vi "ensterMF.vi"() -> ()   [LabVIEW 2019]
uses:
  <vilib>/Utility/error.llb/DialogType.ctl
  <vilib>/DAQmx/write.llb/DAQmx Write (Digital Bool 1Line 1Point).vi
  <vilib>/DAQmx/write.llb/DAQmx Write (Counter Frequency 1Chan 1Samp).vi
  <vilib>/DAQmx/miscellaneous.llb/DAQmx Fill In Error Info.vi
  <vilib>/DAQmx/create/channels.llb/DAQmx Create Channel (CO-Pulse Generation-Frequency).vi
  <vilib>/DAQmx/configure/timing.llb/DAQmx Timing (Implicit).vi
  <vilib>/addons/control/pid/pid.llb/PID (DBL).vi
  <vilib>/Utility/file.llb/Write Delimited Spreadsheet (string).vi
  <instrlib>/Agilent 34970/Agilent 34970.lvlib
  <resource>/objmgr/daqmx.rc
  <vilib>/addons/control/pid/NI_PID_pid.lvlib
  <instrlib>/Yokogawa WT200 Series/Yokogawa WT200 Series.lvlib
panel:
  in  "Tab Control":enum32{"Estufa", "Din", "ET_MF", "TPs", "T_Din"}(tab)
  in  "Ts":dbl=1.0
  out "Time":dbl=300.0 format="%<%H:%M:%S>t"
  in  "STOP":bool
  in  "Idenfier_Estufa":string="medsForno"
  in  "Estufa_ON":bool=TRUE
  in  "Frequency":dbl=1.0 format="%.6f"
  in  "PID gains":T1={"proportional gain (Kc)"=39.6, "integral time (Ti, min)"=14.617, "derivative time (Td, min)"=0.0} {"derivative time (Td, min)" format="%.3f"; "integral time (Ti, min)" format="%.3f"; "proportional gain (Kc)" format="%.6f"}
  out "Process variable and Setpoint":cluster{"initial PV":dbl, "SP:":dbl}(graph)
  out "MV":dbl(graph)
  in  "SP:":dbl(slide)=70.0 min=0.0 max=0.0 scale=25.0..70.0
  out "Temperature CH9 [degC]":dbl
  out "Temperature CH4 [degC]":dbl
  out "Iteration":i32
  out "Duty Cycle":sgl=0.1 min=0.1 max=99.9 format="%#_6f"
  out "PV":dbl
  in  "Tempo de integração (s)":u32=5 min=1 max=60 step=1
  out "Chart tensão numeric":cluster{"V(A)":dbl, "V(B)":dbl, "V(E)":dbl}(graph)={"V(A)"=0.0, "V(B)"=0.0, "V(E)"=228.25999450683594}
  out "Chart corrente numeric":cluster{"I(A)":dbl, "I(B)":dbl, "I(E)":dbl}(graph)={"I(A)"=0.0, "I(B)"=0.0, "I(E)"=0.14239999651908875}
  out "Chart potencia numeric":T2(graph)={"PC(A)"=0.0, "PC(B)"=7.200000254670158e-05, "PC(T)"=7.200000254670158e-05, "PL(A)"=0.0, "PL(B)"=0.0, "PL(T)"=0.0, "PC(E)"=1.0970638990402222, "PL(E)"=1.0099999904632568}
  in  "Realiza medição WT230":bool=TRUE
  in  "Medição contínua? WT230":bool=TRUE
  in  "Parâmetros serial":T3={"Serial VCC"="COM7", "timeout"=2, "baud rate"=600, "flow control"=0, "data bits"=8, "parity"=enum."None", "stop bits"=10, "termination char"=FALSE} {"stop bits" items=["1.0"=10, "1.5"=15, "2.0"=20]; "flow control" items=["None", "XON/XOFF", "RTS/CTS", "XON/XOFF & RTS/CTS", "DTR/DSR", "XON/XOFF & DTR/DSR"]}
  in  "Velocidade (RPM)":u16 min=1000 max=10000 step=100
  in  "Mensagem":T4(ring)=enum."Read power"
  in  "Limite de corrente":dbl=0.075 min=0.0 max=0.4 step=0.01 format="%.4f"
  in  "Limite de tensão":dbl=30.0 min=0.0 max=30.0 step=0.5 format="%.4f"
  in  "Seta carga":bool
  in  "Enviar velocidade":bool
  in  "Envia mensagem":bool
  in  "Parar motor":bool
  out "Tradução":string
  out "Resposta":string
  in  "Liga Fonte":bool
  out "watt num cluster":T5
  out "Corrente de saída":dbl format="%.4f"
  out "Tensão de saída":dbl format="%.4f"
  out "t":dbl
  out "PL(T)":dbl
  out "PC(T)":dbl
  out "PC(E)":dbl
  out "PL(E)":dbl
  in  "Identifier_Watt":string="medsWatt"
  in  "Idenfier_Freio":string="medsFreio"
  out "MV_I":dbl(graph)
  in  "PID gains MF":T1={"proportional gain (Kc)"=83.141, "integral time (Ti, min)"=1.0049, "derivative time (Td, min)"=0.0} {"derivative time (Td, min)" format="%.3f"; "integral time (Ti, min)" format="%.3f"; "proportional gain (Kc)" format="%.6f"}
  out "Grafico MF ENS":cluster{"initial PV":dbl, "SP:":dbl}(graph)
  out "MV_MF":sgl=0.1 min=0.1 max=99.9 format="%#_6f"
  out "PV_MF":dbl
  in  "Ts MF":dbl=1.0
  in  "Automatic":bool
  in  "SP_MF":dbl(slide)=69.0 caption="SP:" min=0.0 max=0.0 scale=25.0..70.0
  in  "Ident_EnsTerMF":string="medsETMF"
  in  "Tab Control 2":enum32{"1-7", "8-15"}(tab)
  out "G. TP 1":cluster{dbl, "index":i32}(graph)
  out "TP 1":dbl
  out "TP 2":dbl
  out "G. TP 2":cluster{dbl, "index":i32}(graph)
  out "G. TP 3":cluster{dbl, "index":i32}(graph)
  out "TP 3":dbl
  out "G. TP 5":cluster{dbl, "index":i32}(graph)
  out "TP 5":dbl
  out "G. TP 6":cluster{dbl, "index":i32}(graph)
  out "TP 6":dbl
  out "G. TP 7":cluster{dbl, "index":i32}(graph)
  out "TP 7":dbl
  out "G. TP 8":cluster{dbl, "index":i32}(graph)
  out "TP 8":dbl
  out "G. TP 10":cluster{dbl, "index":i32}(graph)
  out "TP 10":dbl
  out "G. TP 11":cluster{dbl, "index":i32}(graph)
  out "TP 11":dbl
  out "G. TP 12":cluster{dbl, "index":i32}(graph)
  out "TP 12":dbl
  out "G. TP 13":cluster{dbl, "index":i32}(graph)
  out "TP 13":dbl
  out "G. TP 15":cluster{dbl, "index":i32}(graph)
  out "TP 15":dbl
  in  "Idenfier_Ens. Term.":string="medsETMA"
  out "Chart Temperatura":cluster{dbl, dbl, dbl, dbl, dbl, dbl}(graph)={21.505, 22.941, 24.092, 23.94, 23.972, 20.648}
  out "temperature num cluster":T6
  # "Controle de Temperatura da Estufa"
  # "Geral"
  # "Respostas do Sistema em Malha Fechada"
  # "Controles"
  # "Medidas"
  # "Freio"
  # "Wattímetro WT230 Yokogawa"
  # "Controles:"
  # "Controles"
  # "Medidas"
  # "Respostas temporais"
  # "Medidas"
  # "Inversor de Frequência"
  # "Controles"
  # "Comandos"
  # "Parâmetros Serial"
  # "Controle Automático do Ensaio de Estresse Térmico"
  # "Geral"
  # "Controles"
  # "Medidas"
  # "Temperaturas dos Termopares"
  # "Nome do arquivo:"
  # "Legenda:"
  # "TP 1: Termopar do Capacitor C011"
  # "TP 3: Termopar do Choke L001"
  # "TP 2: Termopar do Capacitor C009"
  # "TP 5: Termopar do Capacitor C006"
  # "TP 6: Termopar do Fusível F002"
  # "TP 7: Termopar do Conector CN204"
  # "TP 8: Termopar do CI SMPS IC 100"
  # "TP 10: Termopar do Indutor L100"
  # "TP 11: Termopar do Capacitor C112"
  # "TP 12: Termopar do Capacitor C504"
  # "TP 13: Termopar do Microcontrolador IC601"
  # "TP 15: Termopar do Dissipador"
  # "Temperaturas do Motor/Freio"
  # "Gráficos:"
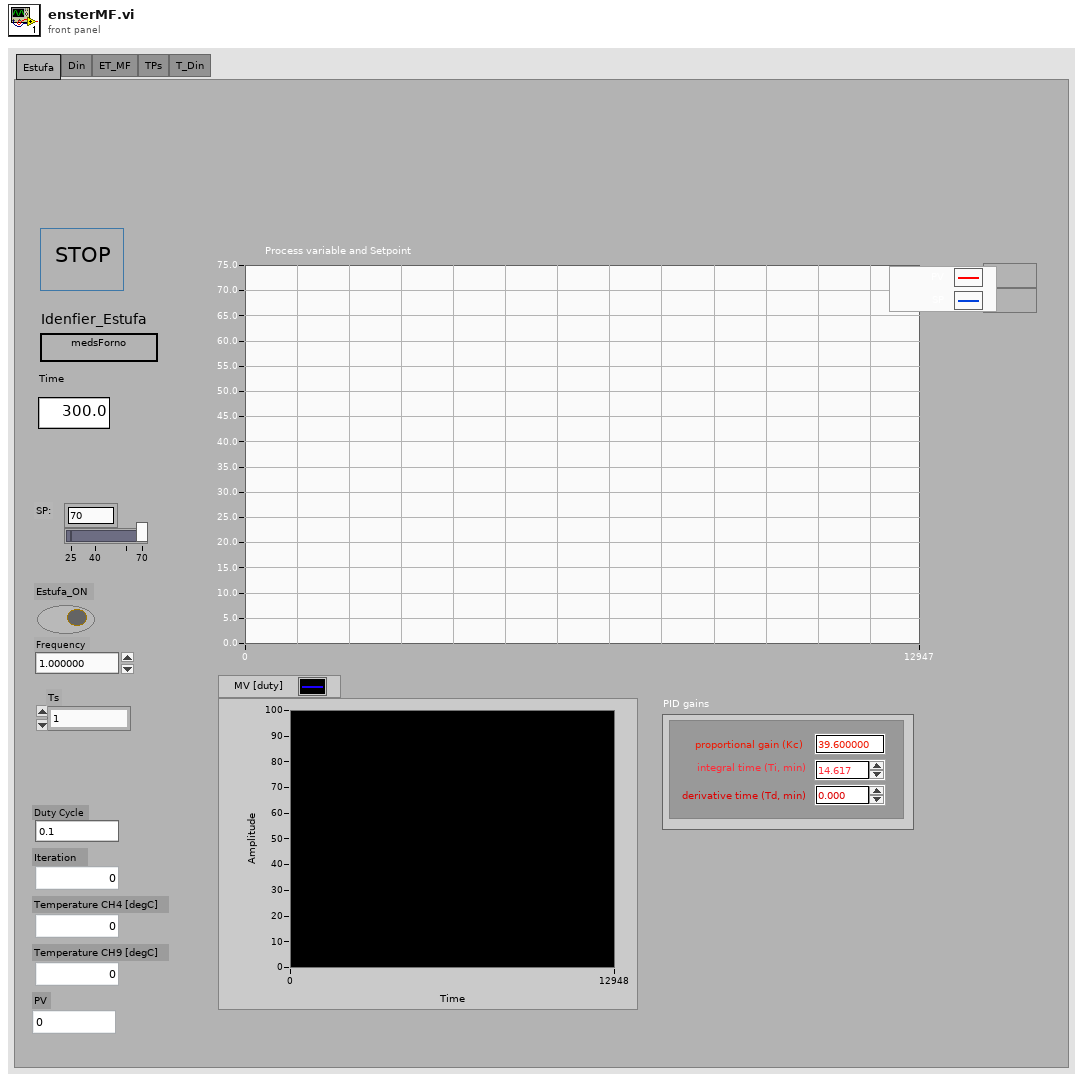
[diagram p1: front panel]
types:
  T1 = cluster{"proportional gain (Kc)":dbl, "integral time (Ti, min)":dbl, "derivative time (Td, min)":dbl}
  T2 = cluster{"PC(A)":dbl, "PC(B)":dbl, "PC(T)":dbl, "PL(A)":dbl, "PL(B)":dbl, "PL(T)":dbl, "PC(E)":dbl, "PL(E)":dbl}
  T3 = cluster{"Serial VCC":refnum<visa-resource-name>, "timeout":u32, "baud rate":u32, "flow control":u16, "data bits":u16, "parity":enum16{"None", "Odd", "Even", "Mark", "Space"}, "stop bits":u16, "termination char":bool}
  T4 = enum16{"Read set speed", "Read operation status", "Read power", "Read starting trials", "Read bus voltage", "Read temperature", "Read power limitation", "Read PWM mode", "Read PWM frequency", "Read real speed"}
  T5 = cluster{"V(A)":dbl, "I(A)":dbl, "V(B)":dbl, "I(B)":dbl, "PC(A)":dbl, "PC(B)":dbl, "PC(T)":dbl, "PL(T)":dbl, "PL(B)":dbl, "PL(A)":dbl, "V(E)":dbl, "PL(E)":dbl, "PC(E)":dbl, "I(E)":dbl, "t":dbl}
  T6 = cluster{"t1 freio":dbl, "t2 bobina":dbl, "t5 bobina":dbl, "t4 estator":dbl, "t3 estator":dbl, "t6 amb":dbl}
  T7 = enum16{"Start Comm.", "End Comm.", "Wait", "Send Static Message", "Set Speed"}
  T8 = enum16{"Thermocouple", "Thermistor", "RTD", "4-Wire RTD", "Default (Last)"}
  T9 = enum8{"Enabled", "Disabled", "Disabled and Grayed Out"}
  T10 = typedef "DialogType.ctl" = u16
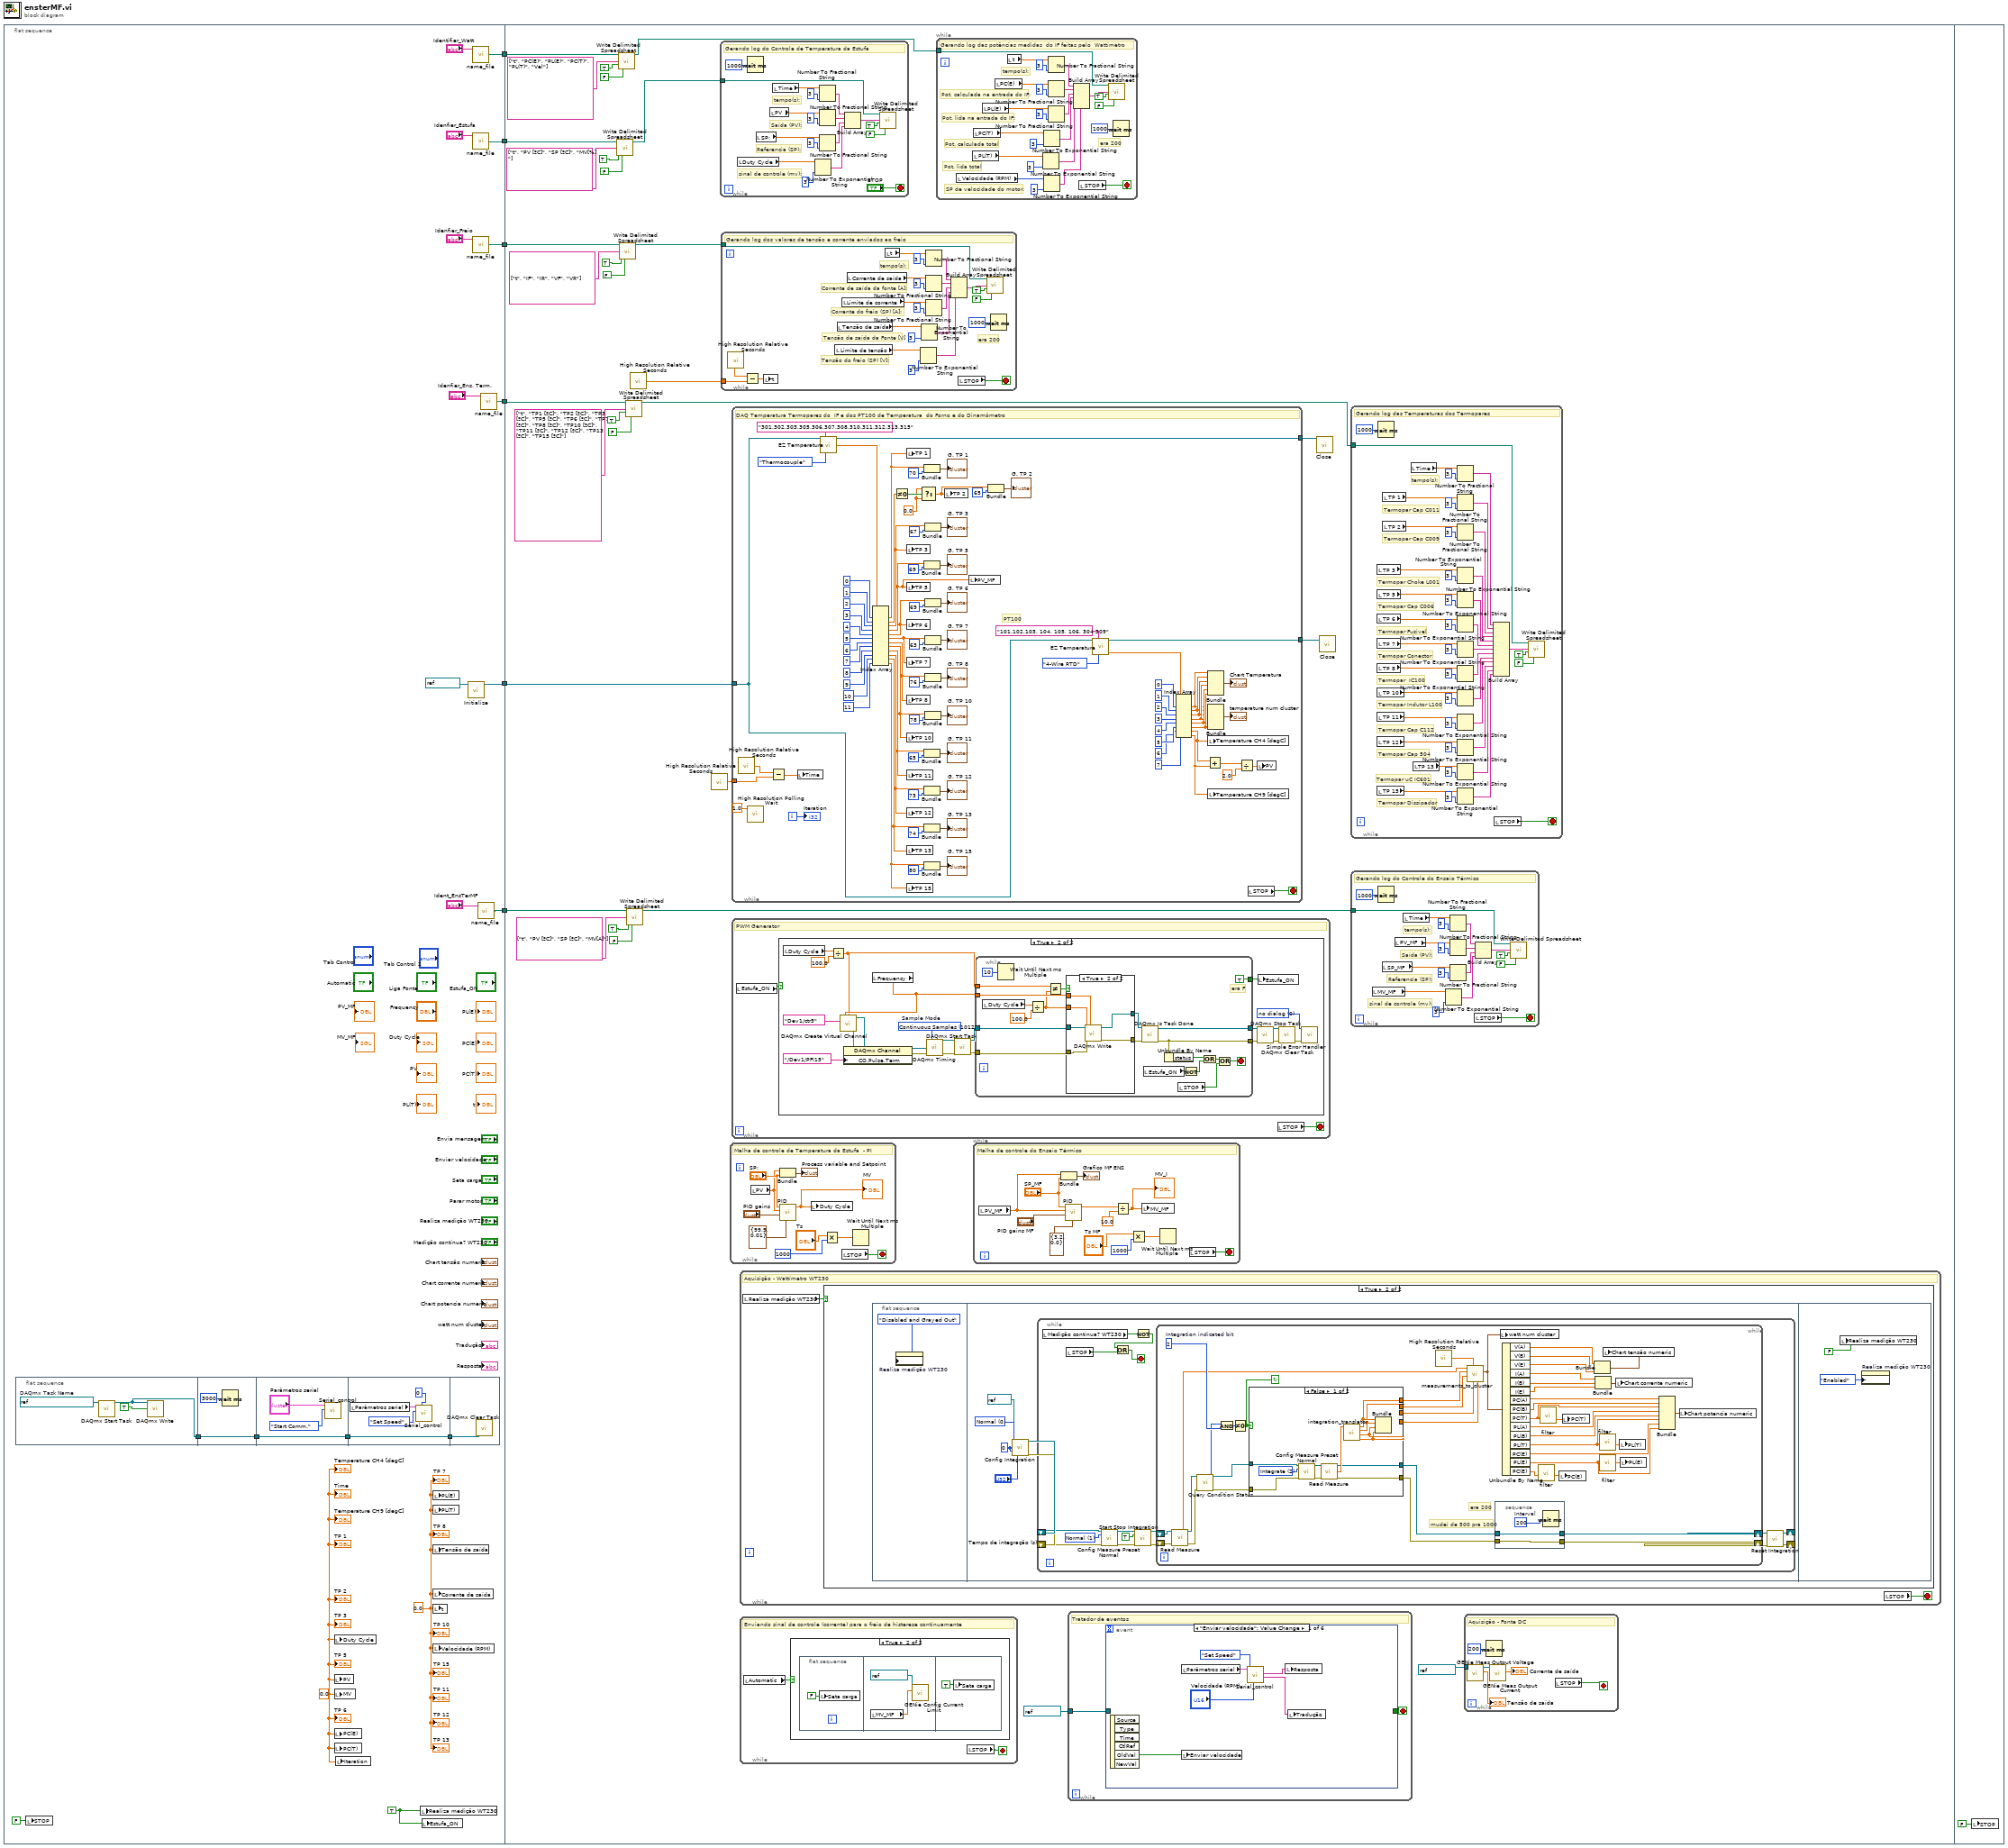
[diagram p0: block diagram]
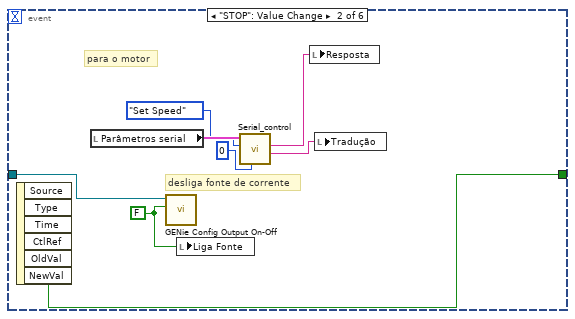
[diagram p3: hidden frame]
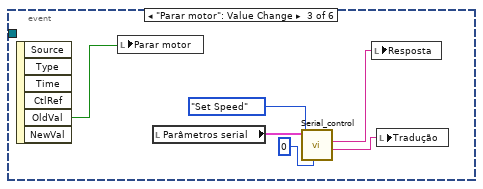
[diagram p4: hidden frame]
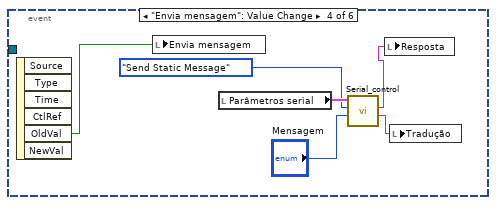
[diagram p5: hidden frame]
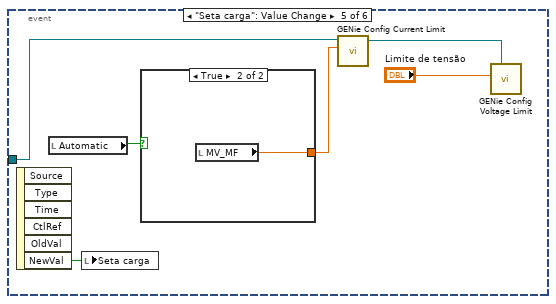
[diagram p6: hidden frame]
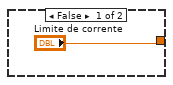
[diagram p7: hidden frame]
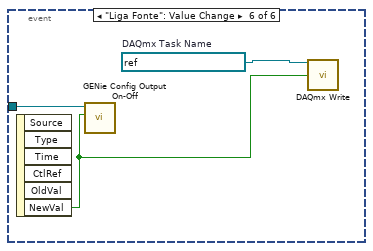
[diagram p8: hidden frame]
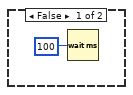
[diagram p9: hidden frame]
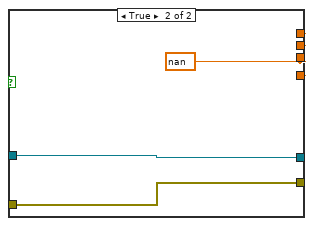
[diagram p10: hidden frame]
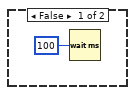
[diagram p11: hidden frame]
diagram:
  n1 = flat-sequence {
    tunnel: [w25] -> w6
    tunnel: [w24] -> w5
    tunnel: [w20] -> w4
    tunnel: [w18] -> w3
    tunnel: [w15] -> w2
    tunnel: [w8] -> w1
    tunnel: w6 -> [w45]
    tunnel: w5 -> [w67]
    tunnel: w4 -> [w64]
    tunnel: w3 -> [w59]
    tunnel: w2 -> [w50]
    tunnel: w1 -> [w41]
    frame #0 {
      w7 = TRUE ("Realiza medição WT230")
      w17 = 0.0 ("Temperature 1")
      w14 = 0.0 ("Temperature 1")
      n2 = flat-sequence {
        tunnel: [w27] -> w13
        tunnel: w13 -> [w30]
        tunnel: [w30] -> w12
        tunnel: w12 -> [w32]
        tunnel: [w32] -> w11
        tunnel: w11 -> [w35]
        tunnel: [w35] -> w10
        tunnel: w10 -> [w39]
        frame #0 {
          w28 = refnum<k21> "alimentacao_inversor"  # DAQmx Task Name
          n3 = call <vilib>:"DAQmx Start Task.vi"("task/channels in"=w28) -> ("task out"=w27:refnum<k21>)  [unwired: 13 in, 1 out]
          n4 = call-poly <vilib>:"DAQmx Write.vi"("task/channels in"=w27, "data"=TRUE) -> ()  [unwired: 11 in, 3 out]
        }
        frame #1 {
          n5 = Wait (ms)(milliseconds to wait=u32 3000) -> ()  [unwired: 1 out]
        }
        frame #2 {
          n6 = call "Serial_control.vi"("Função"=T7."Start Comm.", "comm cluster"="Parâmetros serial") -> ()  [unwired: 3 in, 4 out]
        }
        frame #3 {
          n7 = local read "Parâmetros serial"() -> (w37:T3)
          n8 = call "Serial_control.vi"("Enviar número"=u16 0, "Função"=T7."Set Speed", "comm cluster"=w37) -> ()  [unwired: 2 in, 4 out]
        }
        frame #4 {
          n9 = call <vilib>:"DAQmx Clear Task.vi"("task in"=w39) -> ()  [unwired: 14 in, 1 out]
        }
      }
      n10 = local write "STOP"(FALSE ("STOP")) -> ()
      n11 = local write "Duty Cycle"(w14) -> ()
      n12 = local write "PV"(w14) -> ()
      n13 = local write "MV"(w14) -> ()
      n14 = local write "PC(E)"(w14) -> ()
      n15 = local write "PC(T)"(w14) -> ()
      n16 = local write "Iteration"(w14) -> ()
      n17 = local write "Realiza medição WT230"(w7) -> ()
      n18 = local write "Estufa_ON"(w7) -> ()
      n19 = local write "PL(E)"(w17) -> ()
      n20 = local write "PL(T)"(w17) -> ()
      n21 = local write "Tensão de saída"(w17) -> ()
      n22 = local write "Corrente de saída"(w17) -> ()
      n23 = local write "t"(w17) -> ()
      n24 = local write "Velocidade (RPM)"(w17) -> ()
      n25 = call <instrlib>:"Initialize.vi"("VISA Resource Name"=refnum<visa-resource-name> "Agilent" ("VISA AGILENT")) -> ("VISA Resource Name Out"=w25:refnum<visa-resource-name>)  [unwired: 13 in, 1 out]
      n26 = call "name_file.vi"("Identifier"="Identifier_Watt") -> ("appended path"=w20:path)  [unwired: 2 in]
      n27 = call "name_file.vi"("Identifier"="Idenfier_Estufa") -> ("appended path"=w24:path)  [unwired: 2 in]
      n28 = call "name_file.vi"("Identifier"="Idenfier_Freio") -> ("appended path"=w18:path)  [unwired: 2 in]
      n29 = call "name_file.vi"("Identifier"="Ident_EnsTerMF") -> ("appended path"=w8:path)  [unwired: 2 in]
      n30 = call "name_file.vi"("Identifier"="Idenfier_Ens. Term.") -> ("appended path"=w15:path)  [unwired: 2 in]
      "Temperature CH4 [degC]" <- w14
      "Temperature CH9 [degC]" <- w14
      "Time" <- w14
      "TP 1" <- w14
      "TP 2" <- w14
      "TP 3" <- w14
      "TP 5" <- w14
      "TP 6" <- w14
      "TP 7" <- w17
      "TP 8" <- w17
      "TP 10" <- w17
      "TP 11" <- w17
      "TP 12" <- w17
      "TP 13" <- w17
      "TP 15" <- w17
    }
    frame #1 {
      n31 = call-poly <vilib>:"Write Delimited Spreadsheet.vi"("file path (dialog if empty)"=w67, "1D data"=string[] ["t", "PV [ºC]", "SP [ºC]", "MV[%] "] ("appended array"), "append to file? (new file:F)"=TRUE, "transpose? (no:F)"=FALSE) -> ("new file path (Not A Path if cancelled)"=w68:path)  [unwired: 10 in, 1 out]
      n32 = call-poly <vilib>:"Write Delimited Spreadsheet.vi"("file path (dialog if empty)"=w64, "1D data"=string[] ["t", "PC(E)", "PL(E)", "PC(T)", "PL(T)", "Vel"] ("appended array"), "append to file? (new file:F)"=TRUE, "transpose? (no:F)"=FALSE) -> ("new file path (Not A Path if cancelled)"=w60:path)  [unwired: 10 in, 1 out]
      n33 = call-poly <vilib>:"Write Delimited Spreadsheet.vi"("file path (dialog if empty)"=w59, "1D data"=string[] ["t", "IF", "IR", "VF", "VR"] ("appended array"), "append to file? (new file:F)"=TRUE, "transpose? (no:F)"=FALSE) -> ("new file path (Not A Path if cancelled)"=w55:path)  [unwired: 10 in, 1 out]
      n34 = call-poly <vilib>:"Write Delimited Spreadsheet.vi"("file path (dialog if empty)"=w50, "1D data"=string[] ["t", "TP1 [ºC]", "TP2 [ºC]", "TP3 [ºC]", "TP5 [ºC]", "TP6 [ºC]", "TP7 [ºC]", "TP8 [ºC]", "TP10 [ºC]", "TP11 [ºC]", "TP12 [ºC]", "TP13 [ºC]", "TP15 [ºC]"] ("appended array"), "append to file? (new file:F)"=TRUE, "transpose? (no:F)"=FALSE) -> ("new file path (Not A Path if cancelled)"=w49:path)  [unwired: 10 in, 1 out]
      n35 = call-poly <vilib>:"Write Delimited Spreadsheet.vi"("file path (dialog if empty)"=w41, "1D data"=string[] ["t", "PV [ºC]", "SP [ºC]", "MV[A]"] ("appended array"), "append to file? (new file:F)"=TRUE, "transpose? (no:F)"=FALSE) -> ("new file path (Not A Path if cancelled)"=w40:path)  [unwired: 10 in, 1 out]
      n36 = call <vilib>:"High Resolution Relative Seconds.vi"() -> ("relative seconds"=w54:dbl)
      n37 = call <vilib>:"High Resolution Relative Seconds.vi"() -> ("relative seconds"=w47:dbl)
      n38 = while {
        tunnel: w68 -> [w500]
        stop <- "STOP" stop-if-true
        # "tempo(s):"
        # "Saída (PV):"
        # "Referencia (SP):"
        # "sinal de controle (mv):"
        # "Gerando log do Controle de Temperatura da Estufa"
        n39 = local read "Duty Cycle"() -> (w496:sgl)
        n40 = Wait (ms)(milliseconds to wait=u32 1000) -> ()  [unwired: 1 out]
        n41 = local read "SP:"() -> (w489:dbl)
        n42 = local read "PV"() -> (w495:dbl)
        n43 = local read "Time"() -> (w493:dbl)
        n44 = Number To Exponential String(number=w496, precision (6)=i16 3) -> (E-format string=w498:string)  [unwired: 2 in]
        n45 = Number To Fractional String(number=w493, precision (6)=i16 3) -> (F-format string=w492:string)  [unwired: 2 in]
        n46 = Number To Fractional String(number=w495, precision (6)=i16 3) -> (F-format string=w491:string)  [unwired: 2 in]
        n47 = Number To Fractional String(number=w489, precision (6)=i16 3) -> (F-format string=w487:string)  [unwired: 2 in]
        n48 = Build Array(w492, w491, w487, w498) -> (w488:string[])
        n49 = call-poly <vilib>:"Write Delimited Spreadsheet.vi"("file path (dialog if empty)"=w500, "1D data"=w488, "append to file? (new file:F)"=TRUE, "transpose? (no:F)"=FALSE) -> ()  [unwired: 10 in, 2 out]
      }
      n50 = while {
        tunnel: w55 -> [w261]
        tunnel: w54 -> [w241]
        stop <- w247 stop-if-true
        # "era 200"
        # "Tensão do freio (SP) [V]:"
        # "tempo(s):"
        # "Corrente de saída da fonte [A]:"
        # "Corrente do freio (SP) [A]:"
        # "Tensão de saída da Fonte [V]"
        # "Gerando log dos valores de tensão e corrente enviados ao freio"
        n51 = call <vilib>:"High Resolution Relative Seconds.vi"() -> ("relative seconds"=w242:dbl)
        n52 = Subtract(x=w242, y=w241) -> (x-y=w240:dbl)
        n53 = local write "t"(w240) -> ()
        n54 = local read "Limite de tensão"() -> (w245:dbl)
        n55 = local read "Tensão de saída"() -> (w257:dbl)
        n56 = local read "Limite de corrente"() -> (w250:dbl)
        n57 = local read "Corrente de saída"() -> (w256:dbl)
        n58 = local read "t"() -> (w254:dbl)
        n59 = Number To Exponential String(number=w245, precision (6)=i16 3) -> (E-format string=w243:string)  [unwired: 2 in]
        n60 = Number To Exponential String(number=w257, precision (6)=i16 3) -> (E-format string=w259:string)  [unwired: 2 in]
        n61 = Number To Fractional String(number=w254, precision (6)=i16 3) -> (F-format string=w253:string)  [unwired: 2 in]
        n62 = Number To Fractional String(number=w256, precision (6)=i16 3) -> (F-format string=w252:string)  [unwired: 2 in]
        n63 = Number To Fractional String(number=w250, precision (6)=i16 3) -> (F-format string=w248:string)  [unwired: 2 in]
        n64 = Build Array(w253, w252, w248, w259, w243) -> (w249:string[])
        n65 = local read "STOP"() -> (w247:bool)
        n66 = call-poly <vilib>:"Write Delimited Spreadsheet.vi"("file path (dialog if empty)"=w261, "1D data"=w249, "append to file? (new file:F)"=TRUE, "transpose? (no:F)"=FALSE) -> ()  [unwired: 10 in, 2 out]
        n67 = Wait (ms)(milliseconds to wait=u32 1000) -> ()  [unwired: 1 out]
      }
      n68 = while {
        stop <- w424 stop-if-true
        # "Malha de controle de Temperatura da Estufa  - PI"
        n69 = local read "PV"() -> (w428:dbl)
        n70 = Bundle("PV"=w428, "SP:"="SP:") -> (→"Process variable and Setpoint":cluster{"PV":dbl, "SP:":dbl})  [unwired: 1 in]
        n71 = call-poly <vilib>:"PID.vi"("output range"=cluster{"output high":dbl, "output low":dbl} {"output high"=99.9, "output low"=0.01}, "PID gains"="PID gains", "process variable"=w428, "setpoint"="SP:") -> ("output"=w423:dbl)  [unwired: 6 in, 1 out]
        "MV" <- w423
        n72 = local write "Duty Cycle"(w423) -> ()
        n73 = Multiply(x="Ts", y=u32 1000 ("unsigned 32bit integer")) -> (x*y=w422:dbl)
        n74 = local read "STOP"() -> (w424:bool)
        n75 = Wait Until Next ms Multiple(millisecond multiple=w422) -> ()  [unwired: 1 out]
      }
      n76 = while {
        stop <- w432 stop-if-true
        # "PWM Generator"
        n77 = local read "Estufa_ON"() -> (w433:bool)
        n78 = case shown="True" w433 {
          frame False {
            n79 = Wait (ms)(milliseconds to wait=u32 100) -> ()  [unwired: 1 out]
          }
          frame True {
            w441 = T10 0 items=["no dialog", "OK message", "continue or stop message", "OK message + warnings", "continue/stop + warnings"] ("type of dialog (OK msg:1)")
            w452 = 10123 items=["Finite Samples"=10178, "Continuous Samples"=10123, "Hardware Timed Single Point"=12522]  # Sample Mode
            n80 = local read "Duty Cycle"() -> (w436:sgl)
            n81 = Divide(x=w436, y=100.0) -> (x/y=w435:dbl)
            n82 = local read "Frequency"() -> (w438:dbl)
            n83 = call-poly <vilib>:"DAQmx Create Virtual Channel.vi"("frequency"=w438, "duty cycle"=w435, "counter"=tag "Dev1/ctr3" ("Counter")) -> ("task out"=w455:refnum<k21>, "error out"=w454:errorcluster)  [unwired: 11 in]
            n84 = property class="DAQmx Channel"(reference=w455, error in=w454, "CO.Pulse.Term"=tag "/Dev1/PFI15" ("Output Terminal")) -> (reference out=w451:refnum<k21>, error out=w450:errorcluster)
            n85 = call-poly <vilib>:"DAQmx Timing.vi"("task/channels in"=w451, "sample mode"=w452, "error in"=w450) -> ("task out"=w449:refnum<k21>, "error out"=w448:errorcluster)  [unwired: 11 in]
            n86 = call <vilib>:"DAQmx Start Task.vi"("task/channels in"=w449, "error in"=w448) -> ("task out"=w447:refnum<k21>, "error out"=w446:errorcluster)  [unwired: 12 in]
            n87 = while {
              tunnel: w447 -> [w466]
              tunnel: w446 -> [w464]
              tunnel: [w475] -> w443
              tunnel: [w476] -> w444
              tunnel: [TRUE ("Liga aquecedor")] -> w440
              tunnel: w435 -> [w462]
              tunnel: w438 -> [w460]
              stop <- w469 stop-if-true
              # "era F"
              n88 = local read "Duty Cycle"() -> (w459:sgl)
              n89 = Wait Until Next ms Multiple(millisecond multiple=u32 10) -> ()  [unwired: 1 out]
              n90 = Divide(x=w459, y=100.0) -> (x/y=w457:dbl)
              n91 = Not Equal?(x=w462, y=w457) -> (x != y?=w461:bool)
              n92 = case shown="True" w461 {
                tunnel: [w478 w481] -> w465
                tunnel: w466 -> [w478 w482]
                tunnel: [w477 w483] -> w463
                tunnel: w464 -> [w477 w484]
                tunnel: w457 -> [_ w480]
                tunnel: w460 -> [_ w479]
                frame False {
                }
                frame True {
                  n93 = call-poly <vilib>:"DAQmx Write.vi"("task/channels in"=w482, "frequency"=w479, "duty cycle"=w480, "error in"=w484) -> ("task out"=w481:refnum<k21>, "error out"=w483:errorcluster)  [unwired: 9 in, 1 out]
                }
              }
              n94 = call <vilib>:"DAQmx Is Task Done.vi"("task/channels in"=w465, "error in"=w463) -> ("task out"=w476:refnum<k21>, "error out"=w475:errorcluster)  [unwired: 11 in, 1 out]
              n95 = local read "Estufa_ON"() -> (w472:bool)
              n96 = Unbundle By Name(w475) -> ("status"=w474:bool)
              n97 = local read "STOP"() -> (w467:bool)
              n98 = Not(x=w472) -> (.not. x?=w470:bool)
              n99 = Or(x=w474, y=w470) -> (x .or. y?=w468:bool)
              n100 = Or(x=w468, y=w467) -> (x .or. y?=w469:bool)
            }
            n101 = call <vilib>:"DAQmx Stop Task.vi"("task/channels in"=w444, "error in"=w443) -> ("task out"=w439:refnum<k21>, "error out"=w445:errorcluster)  [unwired: 12 in]
            n102 = local write "Estufa_ON"(w440) -> ()
            n103 = call <vilib>:"DAQmx Clear Task.vi"("task in"=w439, "error in"=w445) -> ("error out"=w442:errorcluster)  [unwired: 13 in]
            n104 = call <vilib>:"Simple Error Handler.vi"("error code (no error:0)"=w441, "error in (no error)"=w442) -> ()  [unwired: 3 in, 5 out]
          }
        }
        n105 = local read "STOP"() -> (w432:bool)
      }
      n106 = while {
        tunnel: [w177] -> w48
        tunnel: w47 -> [w112]
        tunnel: [w111] -> w46
        tunnel: w45 -> [w109]
        i -> [w110]
        stop <- w180 stop-if-true
        w174 = 0.0 ("t")
        # "PT100"
        # "DAQ Temperatura Termopares do  IF e dos PT100 de Temperatura  do Forno e do Dinamômetro"
        n107 = call <vilib>:"High Resolution Relative Seconds.vi"() -> ("relative seconds"=w128:dbl)
        n108 = call <vilib>:"High Resolution Polling Wait.vi"("seconds to wait"=1.0) -> ()  [unwired: 10 in, 1 out]
        n109 = Subtract(x=w128, y=w112) -> (x-y=w124:dbl)
        n110 = local write "Time"(w124) -> ()
        n111 = call <instrlib>:"EZ Temperature.vi"("VISA Resource Name"=w109, "Scan List (empty)"="301,302,303,305,306,307,308,310,311,312,313,315", "Transducer Type (4:Def-Last)"=T8."Thermocouple") -> ("VISA Resource Name Out"=w177:refnum<visa-resource-name>, "Output Array"=w183:dbl[])  [unwired: 10 in, 1 out]
        n112 = Index Array(array=w183, index #1=0 ("index"), index #2=1 ("index"), index #3=2 ("index"), index #4=3 ("index"), index #5=4 ("index"), index #6=5 ("index"), index #7=6 ("index"), index #8=7 ("index"), index #9=8 ("index"), index #10=9 ("index"), index #11=10 ("index"), index #12=11 ("index")) -> (element #1=w173:dbl, element #2=w176:dbl, element #3=w150:dbl, element #4=w108:dbl, element #5=w149:dbl, element #6=w148:dbl, element #7=w147:dbl, element #8=w146:dbl, element #9=w145:dbl, element #10=w144:dbl, element #11=w143:dbl, element #12=w142:dbl)
        n113 = Not Equal To 0?(x=w176) -> (x != 0?=w175:bool)
        n114 = local write "TP 1"(w173) -> ()
        n115 = local write "TP 3"(w150) -> ()
        n116 = local write "TP 5"(w108) -> ()
        n117 = local write "TP 6"(w149) -> ()
        n118 = local write "TP 7"(w148) -> ()
        n119 = local write "TP 8"(w147) -> ()
        n120 = local write "TP 10"(w146) -> ()
        n121 = local write "TP 11"(w145) -> ()
        n122 = local write "TP 12"(w144) -> ()
        n123 = local write "TP 13"(w143) -> ()
        n124 = local write "TP 15"(w142) -> ()
        n125 = Select(t=w174, s=w175, f=w174) -> (s? t:f=w141:dbl)
        n126 = Bundle(w173, "index"=70) -> (→"G. TP 1":cluster{dbl, "index":i32})  [unwired: 1 in]
        n127 = Bundle(w108, "index"=69) -> (→"G. TP 5":cluster{dbl, "index":i32})  [unwired: 1 in]
        n128 = Bundle(w145, "index"=65) -> (→"G. TP 11":cluster{dbl, "index":i32})  [unwired: 1 in]
        n129 = Bundle(w144, "index"=73) -> (→"G. TP 12":cluster{dbl, "index":i32})  [unwired: 1 in]
        n130 = Bundle(w143, "index"=74) -> (→"G. TP 13":cluster{dbl, "index":i32})  [unwired: 1 in]
        n131 = Bundle(w142, "index"=80) -> (→"G. TP 15":cluster{dbl, "index":i32})  [unwired: 1 in]
        n132 = Bundle(w150, "index"=67) -> (→"G. TP 3":cluster{dbl, "index":i32})  [unwired: 1 in]
        n133 = Bundle(w149, "index"=69) -> (→"G. TP 6":cluster{dbl, "index":i32})  [unwired: 1 in]
        n134 = Bundle(w148, "index"=63) -> (→"G. TP 7":cluster{dbl, "index":i32})  [unwired: 1 in]
        n135 = Bundle(w147, "index"=76) -> (→"G. TP 8":cluster{dbl, "index":i32})  [unwired: 1 in]
        n136 = Bundle(w146, "index"=78) -> (→"G. TP 10":cluster{dbl, "index":i32})  [unwired: 1 in]
        n137 = local write "TP 2"(w141) -> ()
        n138 = local write "PV_MF"(w108) -> ()
        n139 = Bundle("t"=w141, "index"=65) -> (→"G. TP 2":cluster{"t":dbl, "index":i32})  [unwired: 1 in]
        n140 = call <instrlib>:"EZ Temperature.vi"("VISA Resource Name"=w109, "Scan List (empty)"="101,102,103, 104, 105, 106, 304,309", "Transducer Type (4:Def-Last)"=T8."4-Wire RTD") -> ("VISA Resource Name Out"=w111:refnum<visa-resource-name>, "Output Array"=w125:dbl[])  [unwired: 10 in, 1 out]
        n141 = Index Array(array=w125, index #1=0 ("index"), index #2=1 ("index"), index #3=2 ("index"), index #4=3 ("index"), index #5=4 ("index"), index #6=5 ("index"), index #7=6 ("index"), index #8=7 ("index")) -> (element #1=w131:dbl, element #2=w132:dbl, element #3=w133:dbl, element #4=w134:dbl, element #5=w135:dbl, element #6=w136:dbl, element #7=w137:dbl, element #8=w138:dbl)
        n142 = Add(x=w137, y=w138) -> (x+y=w126:dbl)
        n143 = Bundle(w131, w132, w133, w134, w135, w136) -> (→"Chart Temperatura":cluster{dbl, dbl, dbl, dbl, dbl, dbl})  [unwired: 1 in]
        n144 = Bundle(w131, w132, w133, w134, w135, w136) -> (→"temperature num cluster":cluster{dbl, dbl, dbl, dbl, dbl, dbl})  [unwired: 1 in]
        n145 = local write "Temperature CH4 [degC]"(w137) -> ()
        n146 = local write "Temperature CH9 [degC]"(w138) -> ()
        n147 = Divide(x=w126, y=2.0) -> (x/y=w127:dbl)
        n148 = local read "STOP"() -> (w180:bool)
        n149 = local write "PV"(w127) -> ()
        "Iteration" <- w110
      }
      n150 = while {
        stop <- w333 stop-if-true
        # "Aquisição - Wattímetro WT230"
        n151 = local read "Realiza medição WT230"() -> (w334:bool)
        n152 = case shown="True" w334 {
          frame False {
            n153 = Wait (ms)(milliseconds to wait=u32 100) -> ()  [unwired: 1 out]
          }
          frame True {
            n154 = flat-sequence {
              frame #0 {
                n155 = property on="Realiza medição WT230" class="Bool (strict)"("DisabledEnum"=T9."Disabled and Grayed Out" ("Disabled")) -> ()  [unwired: 2 in, 2 out]
              }
              frame #1 {
                w339 = u16 0 items=["Normal", "Continuous"] ("Integ Mode (0: Normal)")
                w340 = u32 0 ("Hour (0)")
                n156 = call <instrlib>:"Config Integration.vi"("VISA resource name"=refnum<visa-resource-name> "WT", "Integ Mode (0: Normal)"=w339, "Hour (0)"=w340, "Minute (0)"=w340, "Second (0)"="Tempo de integração (s)") -> ("VISA resource name out"=w342:refnum<visa-resource-name>, "error out"=w341:errorcluster)  [unwired: 9 in]
                n157 = while {
                  shift-right: [w346] -> _
                  shift-left: w342 -> [w344]
                  shift-right: [w345] -> _
                  shift-left: w341 -> [w343]
                  stop <- w347 stop-if-true
                  w353 = u16 1 items=["Clear", "Normal", "Integrate"] ("Preset Pattern (0: Clear)")
                  n158 = local read "Medição contínua? WT230"() -> (w349:bool)
                  n159 = local read "STOP"() -> (w350:bool)
                  n160 = call <instrlib>:"Config Measure Preset Normal.vi"("VISA resource name"=w344, "Preset Pattern (0: Clear)"=w353, "error in (no error)"=w343) -> ("VISA resource name out"=w355:refnum<visa-resource-name>, "error out"=w354:errorcluster)  [unwired: 11 in]
                  n161 = call <instrlib>:"Start Stop Integration.vi"("VISA resource name"=w355, "Start/Stop (F: Stop)"=TRUE, "error in (no error)"=w354) -> ("VISA resource name out"=w358:refnum<visa-resource-name>, "error out"=w357:errorcluster)  [unwired: 11 in]
                  n162 = Not(x=w349) -> (.not. x?=w348:bool)
                  n163 = Or(x=w348, y=w350) -> (x .or. y?=w347:bool)
                  n164 = while {
                    shift-left: w358 -> [w398]
                    shift-right: [w386] -> w352
                    shift-left: w357 -> [w395]
                    shift-right: [w384] -> w351
                    stop <- w394 continue-if-true
                    w401 = u16 2  # Integration indicated bit
                    # "era 200"
                    # "mudei de 500 pra 1000"
                    n165 = call <instrlib>:"Read Measure.vi"("VISA resource name"=w398, "error in (no error)"=w395) -> ("VISA resource name out"=w397:refnum<visa-resource-name>, "Measure Value"=w388:sgl[], "error out"=w396:errorcluster)  [unwired: 10 in, 1 out]
                    n166 = call <instrlib>:"Query Condition Status.vi"("VISA resource name"=w397, "error in (no error)"=w396) -> ("VISA resource name out"=w383:refnum<visa-resource-name>, "Condition"=w399:u16, "error out"=w382:errorcluster)  [unwired: 11 in]
                    n167 = And(x=w399, y=w401) -> (x .and. y?=w400:u16)
                    n168 = Not Equal To 0?(x=w400) -> (x != 0?=w394:bool)
                    n169 = case shown="False" w394 {
                      tunnel: [w412 w419] -> w393
                      tunnel: [w411 w419] -> w392
                      tunnel: [w410 w419] -> w391
                      tunnel: [w409 w419] -> w390
                      tunnel: [w408 w418] -> w387
                      tunnel: [w407 w417] -> w385
                      tunnel: w383 -> [w406 w418]
                      tunnel: w382 -> [w405 w417]
                      frame False {
                        w413 = u16 2 items=["Clear", "Normal", "Integrate"] ("Preset Pattern (0: Clear)")
                        n170 = call <instrlib>:"Config Measure Preset Normal.vi"("VISA resource name"=w406, "Preset Pattern (0: Clear)"=w413, "error in (no error)"=w405) -> ("VISA resource name out"=w416:refnum<visa-resource-name>, "error out"=w415:errorcluster)  [unwired: 11 in]
                        n171 = call <instrlib>:"Read Measure.vi"("VISA resource name"=w416, "error in (no error)"=w415) -> ("VISA resource name out"=w408:refnum<visa-resource-name>, "Measure Value"=w414:sgl[], "error out"=w407:errorcluster)  [unwired: 10 in, 1 out]
                        n172 = call "integration_translator.vi"("Valores integração"=w414) -> ("PI(E)"=w409:sgl, "PI(T)"=w410:sgl, "PI(B)"=w411:sgl, "PI(A)"=w412:sgl)  [unwired: 7 in]
                        n173 = Bundle("PI(A)"=w412, "PI(B)"=w411, "PI(T)"=w410, "PI(E)"=w409) -> ()  [unwired: 1 in, 1 out]
                      }
                      frame True {
                        w419 = nan
                      }
                    }
                    n174 = call <vilib>:"High Resolution Relative Seconds.vi"() -> ("relative seconds"=w389:dbl)
                    n175 = call "measurements_to_cluster.vi"("PI(E)"=w390, "PI(T)"=w391, "relative seconds"=w389, "PI(B)"=w392, "PI(A)"=w393, "Measure Value"=w388) -> ("watt cluster"=w381:T5)  [unwired: 4 in, 1 out]
                    n176 = stacked-sequence {
                      tunnel: w387 -> [w403]
                      tunnel: [w403] -> w386
                      tunnel: w385 -> [w402]
                      tunnel: [w402] -> w384
                      frame #0 {
                        w404 = u32 200  # Interval
                        n177 = Wait (ms)(milliseconds to wait=w404) -> ()  [unwired: 1 out]
                      }
                    }
                    n178 = local write "watt num cluster"(w381) -> ()
                    n179 = Unbundle By Name(w381) -> ("V(A)"=w376:dbl, "V(B)"=w375:dbl, "V(E)"=w374:dbl, "I(A)"=w373:dbl, "I(B)"=w372:dbl, "I(E)"=w371:dbl, "PC(A)"=w370:dbl, "PC(B)"=w369:dbl, "PC(T)"=w368:dbl, "PL(A)"=w366:dbl, "PL(B)"=w365:dbl, "PL(T)"=w364:dbl, "PC(E)"=w363:dbl, "PL(E)"=w362:dbl, "PC(E)"=w360:dbl)
                    n180 = call "filter.vi"("input"=w360) -> ("output"=w359:dbl)  [unwired: 10 in]
                    n181 = call "filter.vi"("input"=w368) -> ("output"=w367:dbl)  [unwired: 10 in]
                    n182 = local write "PC(E)"(w359) -> ()
                    n183 = local write "PC(T)"(w367) -> ()
                    n184 = Bundle("V(A)"=w376, "V(B)"=w375, "V(E)"=w374) -> (w380:cluster{"V(A)":dbl, "V(B)":dbl, "V(E)":dbl})  [unwired: 1 in]
                    n185 = Bundle("I(A)"=w373, "I(B)"=w372, "I(E)"=w371) -> (w379:cluster{"I(A)":dbl, "I(B)":dbl, "I(E)":dbl})  [unwired: 1 in]
                    n186 = call "filter.vi"("input"=w364) -> ("output"=w378:dbl)  [unwired: 10 in]
                    n187 = call "filter.vi"("input"=w362) -> ("output"=w377:dbl)  [unwired: 10 in]
                    n188 = local write "Chart tensão numeric"(w380) -> ()
                    n189 = local write "Chart corrente numeric"(w379) -> ()
                    n190 = local write "PL(T)"(w378) -> ()
                    n191 = local write "PL(E)"(w377) -> ()
                    n192 = Bundle("PC(A)"=w370, "PC(B)"=w369, "PC(T)"=w368, "PL(A)"=w366, "PL(B)"=w365, "PL(T)"=w364, "PC(E)"=w363, "PL(E)"=w362) -> (w361:T2)  [unwired: 1 in]
                    n193 = local write "Chart potencia numeric"(w361) -> ()
                  }
                  n194 = call <instrlib>:"Reset Integration.vi"("VISA resource name"=w352, "error in (no error)"=w351) -> ("VISA resource name out"=w346:refnum<visa-resource-name>, "error out"=w345:errorcluster)  [unwired: 12 in]
                }
              }
              frame #2 {
                n195 = local write "Realiza medição WT230"(FALSE ("Realiza medição")) -> ()
                n196 = property on="Realiza medição WT230" class="Bool (strict)"("DisabledEnum"=T9."Enabled" ("Disabled")) -> ()  [unwired: 2 in, 2 out]
              }
            }
          }
        }
        n197 = local read "STOP"() -> (w333:bool)
      }
      n198 = while {
        stop <- w72 stop-if-true
        # "Enviando sinal de controle (corrente) para o freio de histerese continuamente"
        n199 = local read "Automatic"() -> (w73:bool)
        n200 = case shown="True" w73 {
          frame False {
          }
          frame True {
            n201 = flat-sequence {
              frame #0 {
                n202 = local write "Seta carga"(FALSE ("Seta carga")) -> ()
              }
              frame #1 {
                n203 = local read "MV_MF"() -> (w76:sgl)
                n204 = call <instrlib>:"GENie Config Current Limit.vi"("Current Limit"=w76, "VISA"=refnum<visa-resource-name> "Lambda" ("VISA name")) -> ()  [unwired: 8 in, 2 out]
              }
              frame #2 {
                n205 = local write "Seta carga"(TRUE ("Seta carga")) -> ()
              }
            }
          }
        }
        n206 = local read "STOP"() -> (w72:bool)
      }
      n207 = while {
        tunnel: w60 -> [w285]
        stop <- w271 stop-if-true
        # "era 200"
        # "SP de velocidade do motor:"
        # "Pot. lida total"
        # "tempo(s):"
        # "Pot. calculada na entrada do IF:"
        # "Pot. lida na entrada do IF:"
        # "Pot. calculada total"
        # "Gerando log das potências medidas  do IF feitas pelo  Wattímetro"
        n208 = local read "Velocidade (RPM)"() -> (w267:u16)
        n209 = local read "PL(T)"() -> (w270:dbl)
        n210 = local read "PC(T)"() -> (w281:dbl)
        n211 = local read "PL(E)"() -> (w274:dbl)
        n212 = local read "PC(E)"() -> (w280:dbl)
        n213 = local read "t"() -> (w278:dbl)
        n214 = Number To Exponential String(number=w270, precision (6)=i16 3) -> (E-format string=w268:string)  [unwired: 2 in]
        n215 = Number To Exponential String(number=w281, precision (6)=i16 3) -> (E-format string=w283:string)  [unwired: 2 in]
        n216 = Number To Exponential String(number=w267, precision (6)=i16 3) -> (E-format string=w264:string)  [unwired: 2 in]
        n217 = Number To Fractional String(number=w278, precision (6)=i16 3) -> (F-format string=w277:string)  [unwired: 2 in]
        n218 = Number To Fractional String(number=w280, precision (6)=i16 3) -> (F-format string=w276:string)  [unwired: 2 in]
        n219 = Number To Fractional String(number=w274, precision (6)=i16 3) -> (F-format string=w272:string)  [unwired: 2 in]
        n220 = Build Array(w277, w276, w272, w283, w268, w264) -> (w273:string[])
        n221 = local read "STOP"() -> (w271:bool)
        n222 = call-poly <vilib>:"Write Delimited Spreadsheet.vi"("file path (dialog if empty)"=w285, "1D data"=w273, "append to file? (new file:F)"=TRUE, "transpose? (no:F)"=FALSE) -> ()  [unwired: 10 in, 2 out]
        n223 = Wait (ms)(milliseconds to wait=u32 1000) -> ()  [unwired: 1 out]
      }
      n224 = while {
        stop <- w100 stop-if-true
        # "Malha de controle do Ensaio Térmico"
        n225 = local read "PV_MF"() -> (w104:dbl)
        n226 = Bundle("PV_MF"=w104, "SP_MF"="SP_MF") -> (→"Grafico MF ENS":cluster{"PV_MF":dbl, "SP_MF":dbl})  [unwired: 1 in]
        n227 = call-poly <vilib>:"PID.vi"("output range"=cluster{"output high":dbl, "output low":dbl} {"output high"=3.2, "output low"=0.0}, "PID gains"="PID gains MF", "process variable"=w104, "setpoint"="SP_MF") -> ("output"=w98:dbl)  [unwired: 6 in, 1 out]
        n228 = Divide(x=w98, y=10.0) -> (x/y=w96:dbl)
        "MV_I" <- w96
        n229 = Multiply(x="Ts MF", y=u32 1000 ("unsigned 32bit integer")) -> (x*y=w99:dbl)
        n230 = local write "MV_MF"(w96) -> ()
        n231 = Wait Until Next ms Multiple(millisecond multiple=w99) -> ()  [unwired: 1 out]
        n232 = local read "STOP"() -> (w100:bool)
      }
      n233 = while {
        tunnel: refnum<visa-resource-name> "Lambda" ("VISA name") -> [w294]
        stop <- w295 stop-if-true
        # "Tratador de eventos"
        n234 = event shown="[0] \"Enviar velocidade\": Value Change" {
          selector: _ -> [_ _ _ _ _ _]
          dyn-events: _ -> [_ _ _ _ _ _]
          timeout: _ -> [_ _ _ _ _ _]
          tunnel: w294 -> [_ w303 _ _ w326 w332]
          tunnel: [_ w304 _ _ _ _] -> w295
          event "Enviar velocidade": Value Change {
            n235 = event-data() -> ("OldVal"=w301:bool)  [unwired: 1 in, 5 out]
            n236 = local read "Parâmetros serial"() -> (w300:T3)
            n237 = local write "Enviar velocidade"(w301) -> ()
            n238 = call "Serial_control.vi"("Enviar número"="Velocidade (RPM)", "Função"=T7."Set Speed", "comm cluster"=w300) -> ("translated message"=w297:string, "read buffer"=w298:string)  [unwired: 2 in, 2 out]
            n239 = local write "Resposta"(w298) -> ()
            n240 = local write "Tradução"(w297) -> ()
          }
          event "STOP": Value Change {
            w302 = FALSE ("Output ON")
            # "desliga fonte de corrente"
            # "para o motor"
            n241 = event-data() -> ("NewVal"=w304:bool)  [unwired: 1 in, 5 out]
            n242 = local read "Parâmetros serial"() -> (w309:T3)
            n243 = call <instrlib>:"GENie Config Output On-Off.vi"("Output ON"=w302, "VISA"=w303) -> ()  [unwired: 8 in, 2 out]
            n244 = local write "Liga Fonte"(w302) -> ()
            n245 = call "Serial_control.vi"("Enviar número"=u16 0, "Função"=T7."Set Speed", "comm cluster"=w309) -> ("translated message"=w307:string, "read buffer"=w308:string)  [unwired: 2 in, 2 out]
            n246 = local write "Resposta"(w308) -> ()
            n247 = local write "Tradução"(w307) -> ()
          }
          event "Parar motor": Value Change {
            n248 = event-data() -> ("OldVal"=w312:bool)  [unwired: 1 in, 5 out]
            n249 = local write "Parar motor"(w312) -> ()
            n250 = local read "Parâmetros serial"() -> (w315:T3)
            n251 = call "Serial_control.vi"("Enviar número"=u16 0, "Função"=T7."Set Speed", "comm cluster"=w315) -> ("translated message"=w310:string, "read buffer"=w311:string)  [unwired: 2 in, 2 out]
            n252 = local write "Resposta"(w311) -> ()
            n253 = local write "Tradução"(w310) -> ()
          }
          event "Envia mensagem": Value Change {
            n254 = event-data() -> ("OldVal"=w321:bool)  [unwired: 1 in, 5 out]
            n255 = local write "Envia mensagem"(w321) -> ()
            n256 = local read "Parâmetros serial"() -> (w320:T3)
            n257 = call "Serial_control.vi"("Message"="Mensagem", "Função"=T7."Send Static Message", "comm cluster"=w320) -> ("translated message"=w318:string, "read buffer"=w317:string)  [unwired: 2 in, 2 out]
            n258 = local write "Resposta"(w317) -> ()
            n259 = local write "Tradução"(w318) -> ()
          }
          event "Seta carga": Value Change {
            n260 = event-data() -> ("NewVal"=w322:bool)  [unwired: 1 in, 5 out]
            n261 = local read "Automatic"() -> (w323:bool)
            n262 = local write "Seta carga"(w322) -> ()
            n263 = case shown="True" w323 {
              tunnel: ["Limite de corrente" w329] -> w324
              frame False {
              }
              frame True {
                n264 = local read "MV_MF"() -> (w329:sgl)
              }
            }
            n265 = call <instrlib>:"GENie Config Current Limit.vi"("Current Limit"=w324, "VISA"=w326) -> ("VISA out"=w325:refnum<visa-resource-name>)  [unwired: 8 in, 1 out]
            n266 = call <instrlib>:"GENie Config Voltage Limit.vi"("Volt Limit"="Limite de tensão", "VISA"=w325) -> ()  [unwired: 8 in, 2 out]
          }
          event "Liga Fonte": Value Change {
            w331 = refnum<k21> "resfriamento_freio"  # DAQmx Task Name
            n267 = event-data() -> ("NewVal"=w330:bool)  [unwired: 1 in, 5 out]
            n268 = call <instrlib>:"GENie Config Output On-Off.vi"("Output ON"=w330, "VISA"=w332) -> ()  [unwired: 8 in, 2 out]
            n269 = call-poly <vilib>:"DAQmx Write.vi"("task/channels in"=w331, "data"=w330) -> ()  [unwired: 11 in, 3 out]
          }
        }
      }
      n270 = call <instrlib>:"Close.vi"("VISA Resource Name"=w48) -> ()  [unwired: 14 in, 1 out]
      n271 = call <instrlib>:"Close.vi"("VISA Resource Name"=w46) -> ()  [unwired: 14 in, 1 out]
      n272 = while {
        tunnel: w49 -> [w237]
        stop <- w223 stop-if-true
        # "Termopar Dissipador"
        # "Termopar uC IC601"
        # "Termopar Cap 504"
        # "Termopar Cap C112"
        # "Termopar Indutor L100"
        # "Termopar  IC100"
        # "Termopar Conector"
        # "Termopar Fusivel"
        # "Termopar Cap C006"
        # "tempo(s):"
        # "Termopar Cap C011"
        # "Termopar Cap C009"
        # "Termopar Choke L001"
        # "Gerando log das Temperaturas dos Termopares"
        n273 = local read "TP 3"() -> (w233:dbl)
        n274 = local read "TP 5"() -> (w220:dbl)
        n275 = local read "TP 6"() -> (w219:dbl)
        n276 = local read "TP 7"() -> (w216:dbl)
        n277 = local read "TP 8"() -> (w215:dbl)
        n278 = local read "TP 10"() -> (w212:dbl)
        n279 = local read "TP 11"() -> (w211:dbl)
        n280 = local read "TP 12"() -> (w208:dbl)
        n281 = local read "TP 15"() -> (w205:dbl)
        n282 = Wait (ms)(milliseconds to wait=u32 1000) -> ()  [unwired: 1 out]
        n283 = local read "TP 1"() -> (w222:dbl)
        n284 = local read "TP 2"() -> (w227:dbl)
        n285 = local read "Time"() -> (w231:dbl)
        n286 = local read "TP 13"() -> (w207:dbl)
        n287 = Number To Fractional String(number=w231, precision (6)=i16 3) -> (F-format string=w230:string)  [unwired: 2 in]
        n288 = Number To Fractional String(number=w222, precision (6)=i16 3) -> (F-format string=w229:string)  [unwired: 2 in]
        n289 = Number To Fractional String(number=w227, precision (6)=i16 3) -> (F-format string=w225:string)  [unwired: 2 in]
        n290 = Number To Exponential String(number=w233, precision (6)=i16 3) -> (E-format string=w235:string)  [unwired: 2 in]
        n291 = Number To Exponential String(number=w220, precision (6)=i16 3) -> (E-format string=w204:string)  [unwired: 2 in]
        n292 = Number To Exponential String(number=w219, precision (6)=i16 3) -> (E-format string=w203:string)  [unwired: 2 in]
        n293 = Number To Exponential String(number=w216, precision (6)=i16 3) -> (E-format string=w202:string)  [unwired: 2 in]
        n294 = Number To Exponential String(number=w215, precision (6)=i16 3) -> (E-format string=w201:string)  [unwired: 2 in]
        n295 = Number To Exponential String(number=w212, precision (6)=i16 3) -> (E-format string=w200:string)  [unwired: 2 in]
        n296 = Number To Exponential String(number=w211, precision (6)=i16 3) -> (E-format string=w199:string)  [unwired: 2 in]
        n297 = Number To Exponential String(number=w208, precision (6)=i16 3) -> (E-format string=w198:string)  [unwired: 2 in]
        n298 = Number To Exponential String(number=w207, precision (6)=i16 3) -> (E-format string=w197:string)  [unwired: 2 in]
        n299 = Number To Exponential String(number=w205, precision (6)=i16 3) -> (E-format string=w196:string)  [unwired: 2 in]
        n300 = Build Array(w230, w229, w225, w235, w204, w203, w202, w201, w200, w199, w198, w197, w196) -> (w226:string[])
        n301 = local read "STOP"() -> (w223:bool)
        n302 = call-poly <vilib>:"Write Delimited Spreadsheet.vi"("file path (dialog if empty)"=w237, "1D data"=w226, "append to file? (new file:F)"=TRUE, "transpose? (no:F)"=FALSE) -> ()  [unwired: 10 in, 2 out]
      }
      n303 = while {
        tunnel: w40 -> [w93]
        stop <- w78 stop-if-true
        # "tempo(s):"
        # "Saída (PV):"
        # "Referencia (SP):"
        # "sinal de controle (mv):"
        # "Gerando log do Controle do Ensaio Térmico"
        n304 = local read "MV_MF"() -> (w89:sgl)
        n305 = Wait (ms)(milliseconds to wait=u32 1000) -> ()  [unwired: 1 out]
        n306 = local read "SP_MF"() -> (w82:dbl)
        n307 = local read "PV_MF"() -> (w88:dbl)
        n308 = local read "Time"() -> (w86:dbl)
        n309 = Number To Exponential String(number=w89, precision (6)=i16 3) -> (E-format string=w91:string)  [unwired: 2 in]
        n310 = Number To Fractional String(number=w86, precision (6)=i16 3) -> (F-format string=w85:string)  [unwired: 2 in]
        n311 = Number To Fractional String(number=w88, precision (6)=i16 3) -> (F-format string=w84:string)  [unwired: 2 in]
        n312 = Number To Fractional String(number=w82, precision (6)=i16 3) -> (F-format string=w80:string)  [unwired: 2 in]
        n313 = local read "STOP"() -> (w78:bool)
        n314 = Build Array(w85, w84, w80, w91) -> (w81:string[])
        n315 = call-poly <vilib>:"Write Delimited Spreadsheet.vi"("file path (dialog if empty)"=w93, "1D data"=w81, "append to file? (new file:F)"=TRUE, "transpose? (no:F)"=FALSE) -> ()  [unwired: 10 in, 2 out]
      }
      n316 = while {
        tunnel: refnum<visa-resource-name> "Lambda" ("VISA name") -> [w289]
        stop <- w288 stop-if-true
        # "Aquisição - Fonte DC"
        n317 = call <instrlib>:"GENie Meas Output Voltage.vi"("VISA"=w289) -> ("Output Voltage"=→"Tensão de saída":dbl, "VISA out"=w292:refnum<visa-resource-name>)  [unwired: 8 in, 1 out]
        n318 = Wait (ms)(milliseconds to wait=u32 200) -> ()  [unwired: 1 out]
        n319 = call <instrlib>:"GENie Meas Output Current.vi"("VISA"=w292) -> ("Output Current"=→"Corrente de saída":dbl)  [unwired: 8 in, 2 out]
        n320 = local read "STOP"() -> (w288:bool)
      }
    }
    frame #2 {
      n321 = local write "STOP"(FALSE ("STOP")) -> ()
    }
  }
